vi "close.vi"(8 "error in":errorcluster, 11 "MB_TCP session in":refnum<class "MB_Master_TCP.lvclass">) -> (0 "error out":errorcluster)   [LabVIEW 2025, in "TanksPlcDriver.lvlib"]
uses:
  <vilib>/Plasmionique/MB Master/MB_Master_TCP/MB_Master_TCP.lvclass
  TanksPlcDriver.lvlib
panel:
  # "Tanks  Driver V0.10\nClose"
  # "10.06.2025"
  # "Blaz Kelbl"
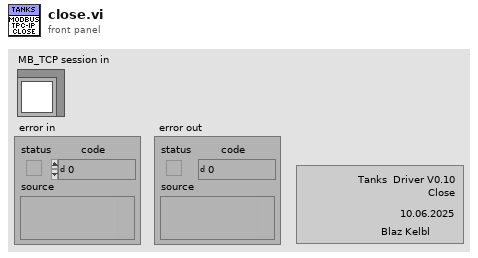
[diagram p1: front panel]
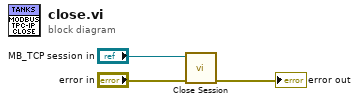
[diagram p0: block diagram]
diagram:
  n1 = call-dynamic "Close Session.vi"("error in (no error)"="error in", "MB TCP session"="MB_TCP session in") -> ("error out"=→"error out":errorcluster)  [unwired: 9 in]
